vi "oax_OrdersStringToDBLArray.vi"(1 "orders to extract":string="Order 1.0") -> (0 "orders to extract out":dbl[](array[numeric])=[1.0] format="%.1g")   [LabVIEW 2017]
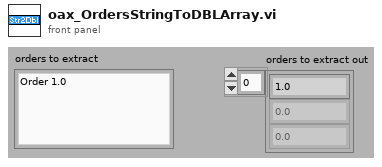
[diagram p1: front panel]
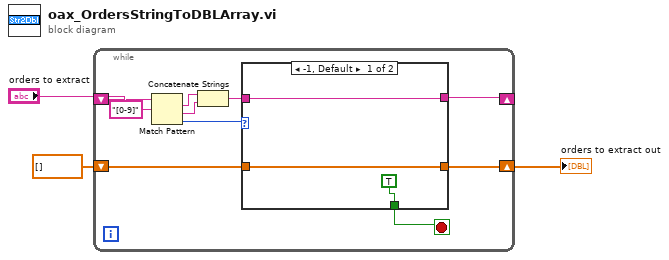
[diagram p0: block diagram]
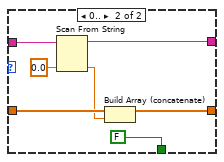
[diagram p2: hidden frame]
diagram:
  n1 = while {
    shift-right: [w4] -> _
    shift-left: "orders to extract" -> [w13]
    shift-right: [w5] -> w2
    shift-left: dbl[] [] ("Orders to extract out") -> [w6]
    stop <- w7 stop-if-true
    n2 = Match Pattern(string=w13, regular expression="[0-9]") -> (match substring=w11:string, after substring=w10:string, offset past match=w9:i32)  [unwired: 1 in, 1 out]
    n3 = Concatenate Strings(w11, w10) -> (w8:string)
    n4 = case shown="-1, Default" w9 {
      tunnel: w8 -> [w15 w22]
      tunnel: [TRUE FALSE] -> w7
      tunnel: w6 -> [w14 w20]
      tunnel: [w14 w18] -> w5
      tunnel: [w15 w17] -> w4
      frame -1, Default {
      }
      frame 0.. {
        n5 = Scan From String(input string=w22, default 1=0.0 ("default value 1")) -> (remaining string=w17:string, output 1=w19:dbl)  [unwired: 3 in, 2 out]
        n6 = Build Array (concatenate)(w20, w19) -> (w18:dbl[])
      }
    }
  }
  "orders to extract out" <- w2
